vi "get channel names from typedef.vi"(8 "error in":errorcluster, 10 "channel classification":T1, 11 "fixed channel configuration":refnum<class "control module configuration.lvclass">) -> (0 "error out":errorcluster, 3 "Channel Names":string[](array[string]))   [LabVIEW 2013, in "control module configuration.lvclass"]
uses:
  control module configuration.lvclass
  <vilib>/NI/Tag Bus Module Framework/channel/channel classification.ctl
  <vilib>/Utility/VariantDataType/VariantType.lvlib
  <vilib>/NI/Tag Bus Module Framework/channel/TBM channel.lvclass
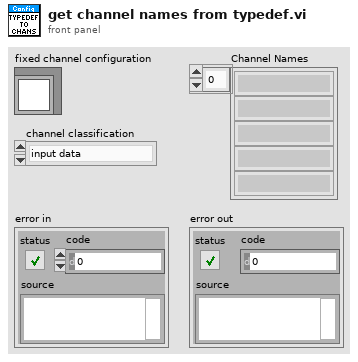
[diagram p1: front panel]
types:
  T1 = typedef "TBM channel.lvclass/channel classification.ctl" = enum16{"input data", "output data", "processing parameter", "processing result"}
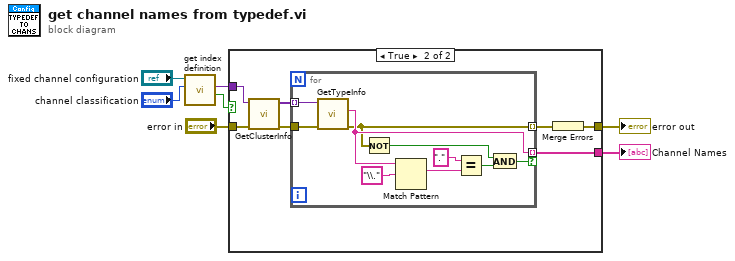
[diagram p0: block diagram]
diagram:
  n1 = call-dynamic "get index definition.vi"("channel classification"="channel classification", "fixed channel configuration in"="fixed channel configuration") -> ("valid?"=w1:bool, "index cluster"=w3:variant)  [unwired: 7 in, 1 out]
  n2 = case shown="True" w1 {
    tunnel: "error in" -> [w8 w13]
    tunnel: [_ w11] -> w6
    tunnel: [w8 w10] -> w4
    tunnel: w3 -> [_ w9]
    frame False {
    }
    frame True {
      n3 = call <vilib>:"GetClusterInfo.vi"("error in (no error)"=w13, "Variant"=w9) -> ("error out"=w14:errorcluster, "Cluster Elements"=w15:variant[])  [unwired: 8 in]
      n4 = for {
        tunnel: w15 -> [w25] mode=indexing
        tunnel: [w22] -> w11 mode=indexing if=w19
        tunnel: w14 -> [w24]
        tunnel: [w17] -> w12 mode=indexing
        n5 = call <vilib>:"GetTypeInfo.vi"("error in (no error)"=w24, "Variant"=w25) -> ("error out"=w17:errorcluster, "Name"=w22:string)  [unwired: 5 in, 3 out]
        n6 = Not(x=w17) -> (.not. x?=w18:bool)
        n7 = Match Pattern(string=w22, regular expression="\\.") -> (match substring=w21:string)  [unwired: 1 in, 3 out]
        n8 = Equal?(x=".", y=w21) -> (x = y?=w16:bool)
        n9 = And(x=w18, y=w16) -> (x .and. y?=w19:bool)
      }
      n10 = Merge Errors(w12) -> (w10:errorcluster)
    }
  }
  "Channel Names" <- w6
  "error out" <- w4
